vi "Layer3_TransmitAndReceiveResponse.vi"(0 "Serial Port to Use":refnum<visa-resource-name>="COM8", 5 "CMD":u16, 7 "Message":string="TestStation1", 9 "Expecting Response":bool=TRUE, 11 "error in (no error)":errorcluster) -> (4 "Serial Port to Use (out)":refnum<visa-resource-name>, 6 "Success":bool, 8 "Response CMD":u16, 10 "Response Message":string, 15 "Error Out":errorcluster)   [LabVIEW 2012]
uses:
  Arduino_Serial_GlobalConstants.vi
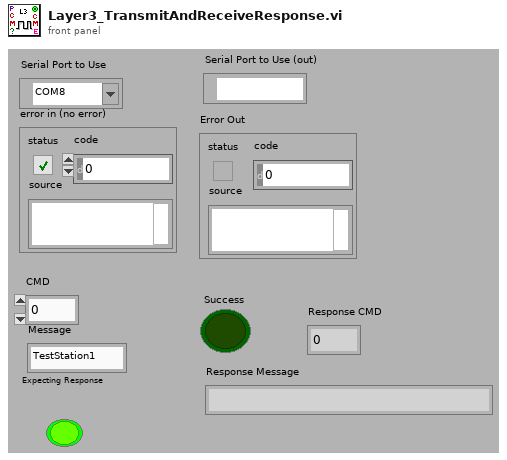
[diagram p1: front panel]
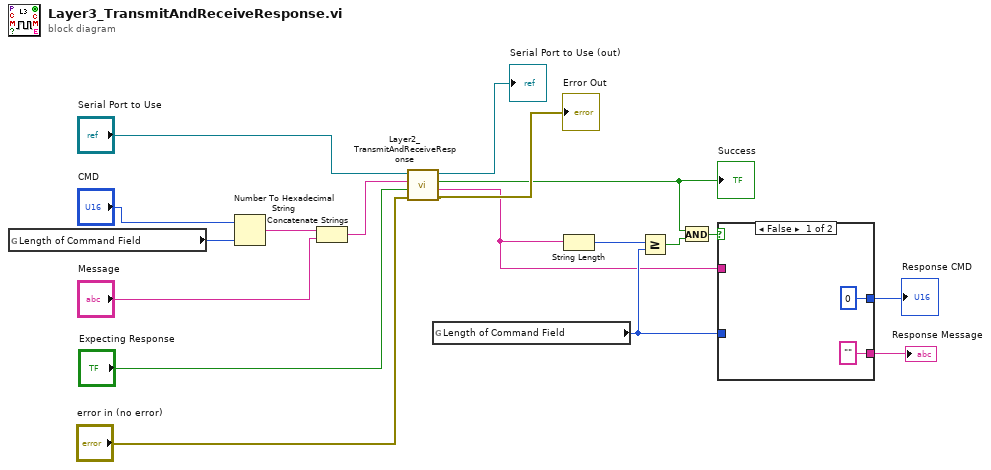
[diagram p0: block diagram]
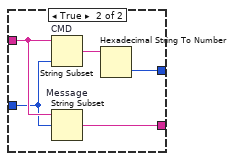
[diagram p2: hidden frame]
diagram:
  n1 = global read "Arduino_Serial_GlobalConstants.vi" "Length of Command Field"() -> (w18:i32)
  n2 = Number To Hexadecimal String(1:w18, 2:"CMD") -> (0:w16:string)
  n3 = Concatenate Strings(w16, "Message") -> (w5:string)
  n4 = call "Layer2_TransmitAndReceiveResponse.vi"("error in (no error)"="error in (no error)", "Expecting Response"="Expecting Response", "Message"=w5, "Serial Port to Use"="Serial Port to Use") -> ("Error Out"=→"Error Out":errorcluster, "Response"=w3:string, "Success"=w4:bool, "Serial Port to Use (out)"=→"Serial Port to Use (out)":refnum<visa-resource-name>)
  "Success" <- w4
  n5 = global read "Arduino_Serial_GlobalConstants.vi" "Length of Command Field"() -> (w11:i32)
  n6 = String Length(string=w3) -> (length=w12:i32)
  n7 = Greater Or Equal?(x=w12, y=w11) -> (x >= y?=w9:bool)
  n8 = And(x=w4, y=w9) -> (x .and. y?=w10:bool)
  n9 = case shown="False" w10 {
    tunnel: w3 -> [_ w24]
    tunnel: w11 -> [_ w23]
    tunnel: [u32 0 w22] -> w14
    tunnel: ["" ("Layer2 Payload") w21] -> w13
    frame False {
    }
    frame True {
      n10 = String Subset "CMD"(string=w24, length (rest)=w23) -> (substring=w25:string)  [unwired: 1 in]
      n11 = String Subset "Message"(string=w24, offset (0)=w23) -> (substring=w21:string)  [unwired: 1 in]
      n12 = Hexadecimal String To Number(string=w25) -> (number=w22:u32)  [unwired: 2 in, 1 out]
    }
  }
  "Response Message" <- w13
  "Response CMD" <- w14
